vi "Instr_InitObject.vi"(8 "error in (no error)":errorcluster, 9 "Instrument Configuration":variant, 10 "GPIB Address":string, 11 "Pickering in":refnum<class "Pickering.lvclass">) -> (0 "error out":errorcluster, 3 "Pickering out":refnum<class "Pickering.lvclass">)   [LabVIEW 2013, in "Pickering.lvclass"]
uses:
  Pickering.lvclass
  InstrumentSetup.vi
  PickeringMUX_CommandsGlobal.vi
  PickeringMatrix_CommandsGlobal.vi
  InstrControl.lvclass
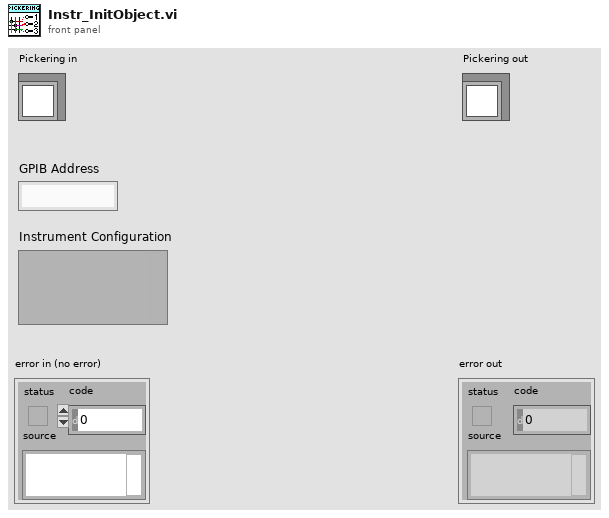
[diagram p1: front panel]
types:
  T1 = cluster{"Matrix address":string, "Mux1 address":string, "Mux2 address":string, "Matrix used?":bool, "Pickering":refnum<class "Pickering.lvclass">, "Matrix X Channels":cluster{"Bias Supply / SMU LO":i32, "Bias Supply / SMU HI":i32, "CV Box LO":i32, "CV Box HI":i32, "CV Box LO IN":i32, "CV Box HI IN":i32, "Volt meter LO":i32, "Volt meter HI":i32, "Mux1 C1":i32, "Mux1 C2":i32, "Mux2 C1":i32, "Mux2 C2":i32}}
  T2 = cluster{"Matrix address":string, "Instrument name":string, "Instrument type":u16, "Command \"Matrix Reset\"":string, "Command \"Connect Matrix Channels\"":string, "Command \"Disconnect Matrix Channels\"":string}
  T3 = cluster{"Mux1 address":string, "Mux2 address":string, "Instrument name":string, "Instrument type":u16, "Command \"MUX Reset\"":string, "Command \"Select MUX Channel\"":string}
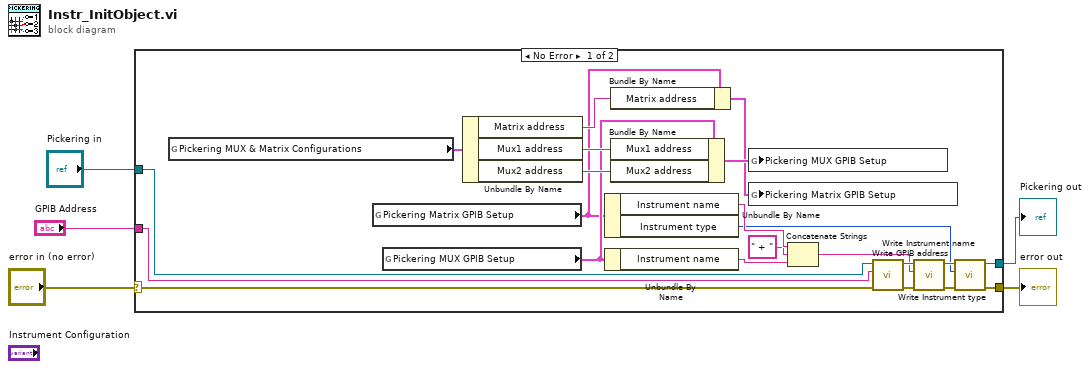
[diagram p0: block diagram]
diagram:
  n1 = case shown="No Error" "error in (no error)" {
    selector: "error in (no error)" -> [w22 w29]
    tunnel: [w15 w29] -> w1
    tunnel: "Pickering in" -> [w21 w28]
    tunnel: [w14 w28] -> w2
    tunnel: "GPIB Address" -> [w10 _]
    frame No Error {
      n2 = global read "InstrumentSetup.vi" "Pickering MUX & Matrix Configurations"() -> (w27:T1)
      n3 = global read "PickeringMatrix_CommandsGlobal.vi" "Pickering Matrix GPIB Setup"() -> (w8:T2)
      n4 = global read "PickeringMUX_CommandsGlobal.vi" "Pickering MUX GPIB Setup"() -> (w9:T3)
      n5 = Unbundle By Name(w27) -> ("Matrix address"=w13:string, "Mux1 address"=w12:string, "Mux2 address"=w11:string)
      n6 = Unbundle By Name(w8) -> ("Instrument name"=w20:string, "Instrument type"=w16:u16)
      n7 = Unbundle By Name(w9) -> ("Instrument name"=w19:string)
      n8 = Bundle By Name(cluster=w8, "Matrix address"=w13) -> (w6:T2)
      n9 = Bundle By Name(cluster=w9, "Mux1 address"=w12, "Mux2 address"=w11) -> (w7:T3)
      n10 = global write "PickeringMUX_CommandsGlobal.vi" "Pickering MUX GPIB Setup"(w7) -> ()
      n11 = global write "PickeringMatrix_CommandsGlobal.vi" "Pickering Matrix GPIB Setup"(w6) -> ()
      n12 = Concatenate Strings(w20, " + ", w19) -> (w17:string)
      n13 = call-dynamic "Write GPIB address.vi"("error in (no error)"=w22, "GPIB address"=w10, "InstControl in"=w21) -> ("error out"=w24:errorcluster, "InstControl out"=w26:refnum<class "Pickering.lvclass">)  [unwired: 7 in]
      n14 = call-dynamic "Write Instrument name.vi"("error in (no error)"=w24, "Instrument name"=w17, "InstControl in"=w26) -> ("error out"=w23:errorcluster, "InstControl out"=w25:refnum<class "Pickering.lvclass">)  [unwired: 7 in]
      n15 = call-dynamic "Write Instrument type.vi"("error in (no error)"=w23, "Instrument type"=w16, "InstControl in"=w25) -> ("error out"=w15:errorcluster, "InstControl out"=w14:refnum<class "Pickering.lvclass">)  [unwired: 7 in]
    }
    frame Error {
    }
  }
  "error out" <- w1
  "Pickering out" <- w2
